vi "Open.vi"(8 "error in":errorcluster, 9 "Editable":bool, 10 "Path":path) -> (0 "error out":errorcluster, 3 "SpreadsheetDoc":refnum<k24>, 5 "Stream":refnum<k24>)   [LabVIEW 2019, in "Open Xml.lvlib"]
uses:
  Open Xml.lvlib
  D:/git/Open-Xml-LabVIEW/Source/DocumentFormat.OpenXml.dll
  DocumentFormat.OpenXml.dll
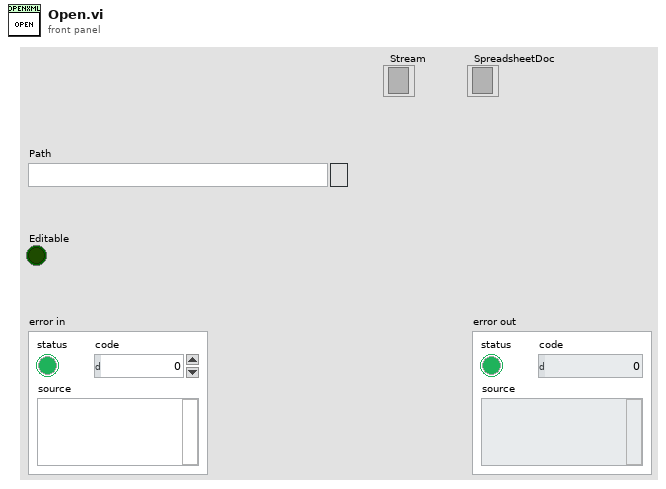
[diagram p1: front panel]
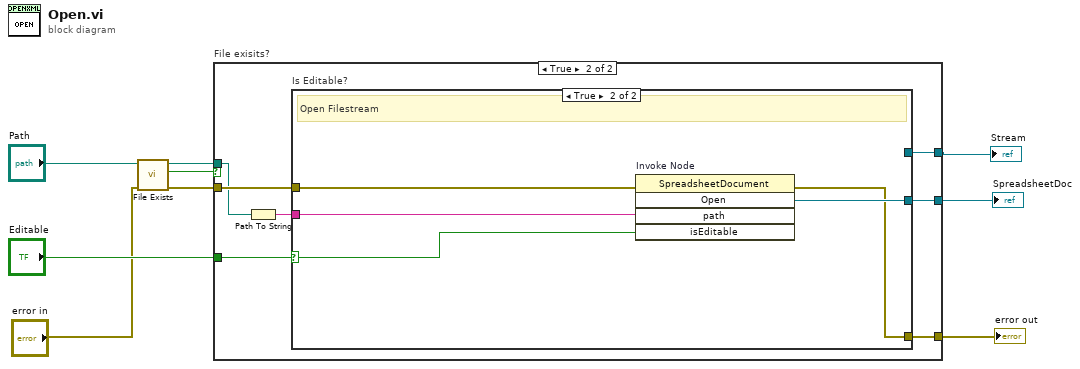
[diagram p0: block diagram]
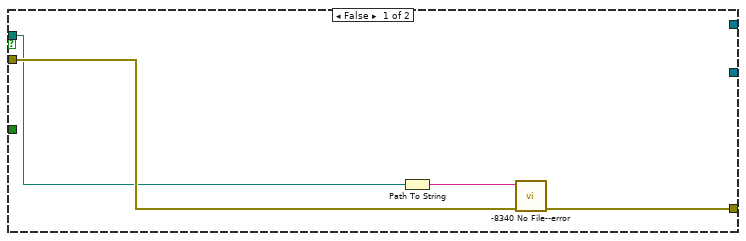
[diagram p2: hidden frame]
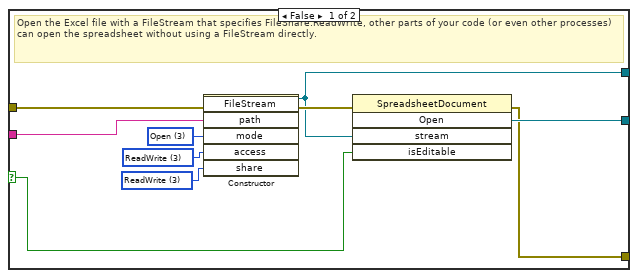
[diagram p3: hidden frame]
diagram:
  n1 = call "File Exists.vi"("error in"="error in", "File Path"="Path") -> ("error out"=w5:errorcluster, "Exists"=w7:bool, "File Path (dup)"=w6:path)  [unwired: 7 in]
  n2 = case "File exisits?" shown="True" w7 {
    tunnel: "Editable" -> [_ w20]
    tunnel: w6 -> [w11 w16]
    tunnel: w5 -> [w13 w19]
    tunnel: [w12 w17] -> w2
    tunnel: [_ w18] -> w4
    tunnel: [_ w14] -> w1
    frame False {
      n3 = Path To String(path=w11) -> (string=w10:string)
      n4 = call "-8340 No File--error.vi"("error in (no error)"=w13, "File Path"=w10) -> ("error out"=w12:errorcluster)  [unwired: 8 in, 1 out]
    }
    frame True {
      n5 = Path To String(path=w16) -> (string=w15:string)
      n6 = case "Is Editable?" shown="True" w20 {
        selector: w20 -> [w29 w35]
        tunnel: w19 -> [w27 w34]
        tunnel: [w30 w33] -> w18
        tunnel: [w22 w32] -> w17
        tunnel: w15 -> [w28 w31]
        tunnel: [w21 _] -> w14
        frame False {
          w23 = 3 items=["None"=0, "Read"=1, "Write"=2, "ReadWrite"=3, "Delete"=4, "Inheritable"=16] ("share")
          w24 = 3 items=["Read"=1, "Write"=2, "ReadWrite"=3] ("access")
          w25 = 3 items=["CreateNew"=1, "Create"=2, "Open"=3, "OpenOrCreate"=4, "Truncate"=5, "Append"=6] ("mode")
          # "Open the Excel file with a FileStream that specifies FileShare.ReadWrite, other parts of your code (or even other processes) can open the spreadsheet without using a FileStream directly."
          n7 = constructor class="FileStream"(error in=w27, "path"=w28, "mode"=w25, "access"=w24, "share"=w23) -> (reference out=w21:refnum<k24>, error out=w26:errorcluster)  [unwired: 2 in, 5 out]
          n8 = invoke on="Invoke Node" class="SpreadsheetDocument" method="Open"(error in=w26, "stream"=w21, "isEditable"=w29) -> (error out=w22:errorcluster, "Open"=w30:refnum<k24>)  [unwired: 2 in, 3 out]
        }
        frame True {
          # "Open Filestream"
          n9 = invoke on="Invoke Node" class="SpreadsheetDocument" method="Open"(error in=w34, "path"=w31, "isEditable"=w35) -> (error out=w32:errorcluster, "Open"=w33:refnum<k24>)  [unwired: 2 in, 3 out]
        }
      }
    }
  }
  "SpreadsheetDoc" <- w4
  "error out" <- w2
  "Stream" <- w1
